vi "Victor linearize.vi"(8 "Deadband":dbl=0.082, 11 "Input":dbl) -> (3 "Output":dbl)   [LabVIEW 2012]
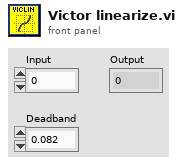
[diagram p1: front panel]
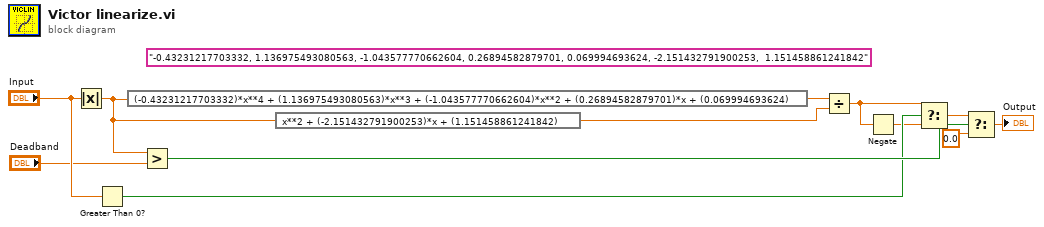
[diagram p0: block diagram]
diagram:
  (unwired) "-0.43231217703332, 1.136975493080563, -1.043577770662604, 0.26894582879701, 0.069994693624, -2.151432791900253,  1.151458861241842"
  n1 = Absolute Value(x="Input") -> (abs(x)=w7:dbl)
  n2 = Greater Than 0?(x="Input") -> (x > 0?=w4:bool)
  n3 = expression code="(-0.43231217703332)*x**4 + (1.136975493080563)*x**3 + (-1.043577770662604)*x**2 + (0.26894582879701)*x + (0.069994693624)"(w7) -> (w11:dbl)
  n4 = Greater?(x=w7, y="Deadband") -> (0:w9:bool)
  n5 = expression code="x**2 + (-2.151432791900253)*x + (1.151458861241842)"(w7) -> (w12:dbl)
  n6 = Divide(x=w11, y=w12) -> (x/y=w2:dbl)
  n7 = Negate(x=w2) -> (-x=w3:dbl)
  n8 = Select(t=w2, s=w4, f=w3) -> (s? t:f=w6:dbl)
  n9 = Select(t=w6, s=w9, f=0.0) -> (s? t:f=→"Output":dbl)
